vi "扫描曲线生成.vi"(7 "坐标轴映射":T1, 9 "Y":dbl[](array[numeric]), 11 "X":dbl[](array[numeric])) -> (3 "曲线":cluster{dbl[], dbl[]}[](array[cluster]), 5 "突变电压":i32)   [LabVIEW 2021]
uses:
  <vilib>/Analysis/NI_AALPro.lvlib
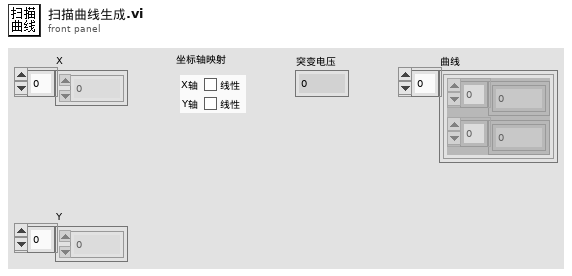
[diagram p1: front panel]
types:
  T1 = typedef "坐标轴映射.ctl" = cluster{"X轴":bool, "Y轴":bool}
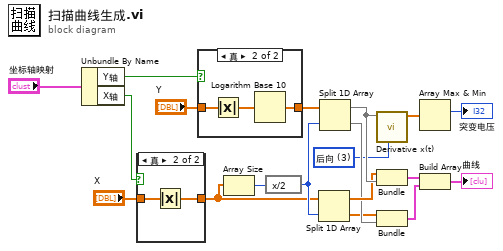
[diagram p0: block diagram]
diagram:
  w5 = u16 3 items=["二阶中心", "四阶中心", "前向", "后向"] ("method")
  n1 = Unbundle By Name("坐标轴映射") -> ("Y轴"=w3:bool, "X轴"=w1:bool)
  n2 = case shown="真" w1 {
    tunnel: "X" -> [w20 w22]
    tunnel: [w20 w21] -> w2
    frame False {
    }
    frame True {
      n3 = Absolute Value(x=w22) -> (abs(x)=w21:dbl[])
    }
  }
  n4 = case shown="真" w3 {
    tunnel: "Y" -> [w23 w26]
    tunnel: [w23 w24] -> w16
    frame False {
    }
    frame True {
      n5 = Absolute Value(x=w26) -> (abs(x)=w25:dbl[])
      n6 = Logarithm Base 10(1:w25) -> (0:w24:dbl[])
    }
  }
  n7 = Array Size(array=w2) -> (size(s)=w17:i32)
  n8 = expression code="x/2"(w17) -> (w18:i32)
  n9 = Split 1D Array(array=w2, index=w18) -> (first subarray=w15:dbl[], second subarray=w13:dbl[])
  n10 = Split 1D Array(array=w16, index=w18) -> (first subarray=w19:dbl[], second subarray=w14:dbl[])
  n11 = call <vilib>:"Derivative x(t).vi"("method"=w5, "X"=w19) -> ("dX/dt"=w6:dbl[])  [unwired: 8 in, 1 out]
  n12 = Bundle(w15, w19) -> (w11:cluster{dbl[], dbl[]})  [unwired: 1 in]
  n13 = Bundle(w13, w14) -> (w12:cluster{dbl[], dbl[]})  [unwired: 1 in]
  n14 = Array Max & Min(array=w6) -> (max index (indices)=→"突变电压":i32)  [unwired: 3 out]
  n15 = Build Array(w11, w12) -> (→"曲线":cluster{dbl[], dbl[]}[])
